vi "Configure Duty Cycle.vi"(6 "Reference Value (50%)":dbl=50.0 format="%#_4g", 8 "error in (no error)":errorcluster, 9 "Reference Type (0:Percent)":i32(ring) items=["Percent", "Volts"], 11 "VISA resource name":refnum<visa-resource-name>) -> (0 "error out":errorcluster, 3 "VISA resource name out":refnum<visa-resource-name>)   [LabVIEW 2020, in "Counter.lvlib" / "PICOTEST U62XXA series.lvlib"]
doc: "Configures the settings required for Duty Cycle measurements. Duty Cycle measurements can only be taken at channel 1.\n\n<B>Note:</B>\nThe U6220A model <B>does not</B> support the \"Duty Cycle\" commands.\n\nThe measurement arming is coupled to Auto. Arming can be changed by calling any of the Arming VIs."
uses:
  PICOTEST U62XXA series.lvlib
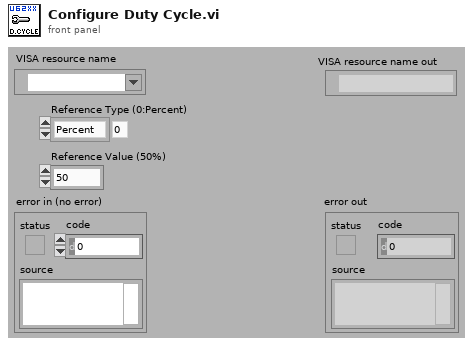
[diagram p1: front panel]
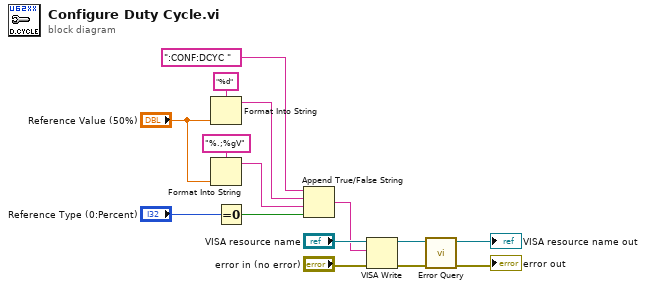
[diagram p0: block diagram]
diagram:
  n1 = Format Into String(format string="%d", "Reference Value (50%)") -> (resulting string=w8:string)  [unwired: 2 in, 1 out]
  n2 = Format Into String(format string="%.;%gV", "Reference Value (50%)") -> (resulting string=w9:string)  [unwired: 2 in, 1 out]
  n3 = Equal To 0?(x="Reference Type (0:Percent)") -> (x = 0?=w12:bool)
  n4 = Append True/False String(1:w12, 2:w9, 3:w8, 4:":CONF:DCYC " ("format string")) -> (0:w6:string)
  n5 = VISA Write(VISA resource name="VISA resource name", write buffer=w6, error in (no error)="error in (no error)") -> (VISA resource name out=w5:refnum<visa-resource-name>, error out=w3:errorcluster)  [unwired: 1 out]
  n6 = call "Error Query.vi"("error in (no error)"=w3, "VISA resource name"=w5) -> ("error out"=→"error out":errorcluster, "VISA resource name out"=→"VISA resource name out":refnum<visa-resource-name>)  [unwired: 6 in, 2 out]
